vi "metronome.vi"(8 "error in (no error)":errorcluster, 11 "Refnum in":T1) -> (0 "error out":errorcluster)   [LabVIEW 2014]
uses:
  Controls/FPGA Reference.ctl
  Controls/Application Data.vi
  <vilib>/Utility/error.llb/Error Cluster From Error Code.vi
  <vilib>/rvi/errors/niLvFpgaAdjustHostInterfaceError.vi
  <vilib>/rvi/interface/nirviReadWriteControl/nirviReadWriteControl.xnode
  <vilib>/rvi/interface/Simulation/niFpgaSimulationCallBeginRW.vi
  NiFpgaLv.dll
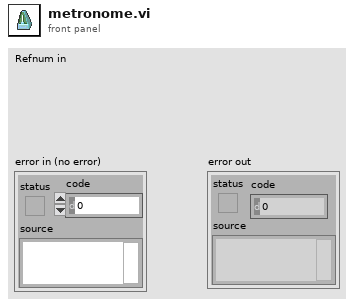
[diagram p1: front panel]
types:
  T1 = typedef "FPGA Reference.ctl" = refnum<k20>
  T2 = cluster{"LED 0":bool, "LED 1":bool, "LED 2":bool, "LED 3":bool}
  T3 = typedef "playback state.ctl" = enum16{"Load File", "Save File", "Play", "Record", "Stop", "Rewind"}
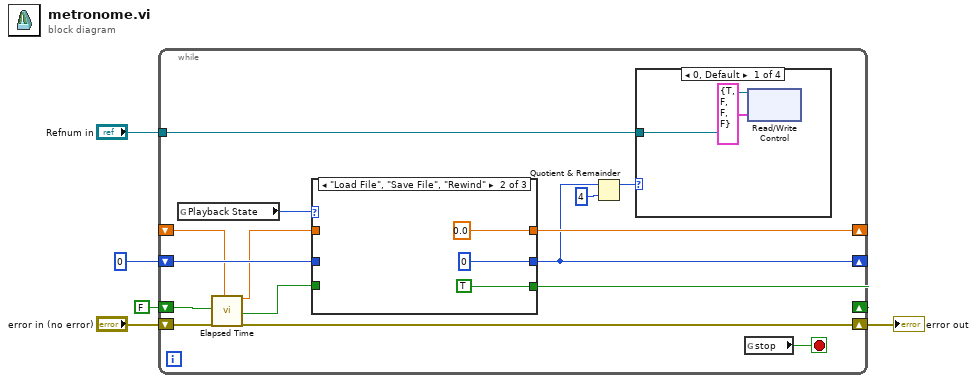
[diagram p0: block diagram]
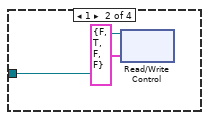
[diagram p2: hidden frame]
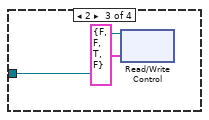
[diagram p3: hidden frame]
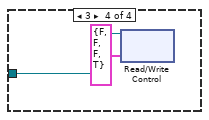
[diagram p4: hidden frame]
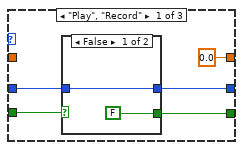
[diagram p5: hidden frame]
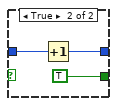
[diagram p6: hidden frame]
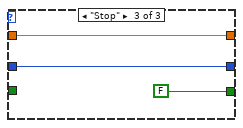
[diagram p7: hidden frame]
diagram:
  n1 = while {
    shift-right: [w11] -> _
    shift-left: 0 -> [w17]
    shift-right: [w16] -> _
    shift-left: FALSE -> [w15]
    shift-right: [w13] -> _
    shift-left: _ -> [w12]
    tunnel: "Refnum in" -> [w8]
    shift-right: [w6] -> w2
    shift-left: "error in (no error)" -> [w7]
    stop <- w20 stop-if-true
    n2 = global read "Application Data.vi" "Playback State"() -> (w19:T3)
    n3 = call "Elapsed Time"("Reset"=w15, "error in (no error)"=w7, "Set Start Time (s)"=w12) -> ("Present (s)"=w14:dbl, "Time has Elapsed"=w18:bool, "error out"=w6:errorcluster)  [unwired: 9 in, 5 out]
    n4 = case shown="\"Load File\", \"Save File\", \"Rewind\"" w19 {
      tunnel: w18 -> [w31 _ _]
      tunnel: w17 -> [w33 _ w42]
      tunnel: [w32 0 w42] -> w11
      tunnel: [w30 TRUE FALSE] -> w16
      tunnel: w14 -> [_ _ w44]
      tunnel: [0.0 ("Present (s)") 0.0 ("Present (s)") w44] -> w13
      frame "Play", "Record" {
        n5 = case shown="False" w31 {
          tunnel: w33 -> [w35 w38]
          tunnel: [w35 w37] -> w32
          tunnel: [FALSE TRUE] -> w30
          frame False {
          }
          frame True {
            n6 = Increment(x=w38) -> (x+1=w37:i32)
          }
        }
      }
      frame "Load File", "Save File", "Rewind" {
      }
      frame "Stop" {
      }
    }
    n7 = Quotient & Remainder(x=w11, y=4) -> (x-y*floor(x/y)=w9:i32)  [unwired: 1 out]
    n8 = case shown="0, Default" w9 {
      tunnel: w8 -> [w22 w24 w26 w28]
      frame 0, Default {
        n9 = xnode "Read/Write Control"("FPGA VI Reference In"=w22, "LEDs"=T2 {"LED 0"=TRUE, "LED 1"=FALSE, "LED 2"=FALSE, "LED 3"=FALSE}) -> ()  [unwired: 1 in, 2 out]
      }
      frame 1 {
        n10 = xnode "Read/Write Control"("FPGA VI Reference In"=w24, "LEDs"=T2 {"LED 0"=FALSE, "LED 1"=TRUE, "LED 2"=FALSE, "LED 3"=FALSE}) -> ()  [unwired: 1 in, 2 out]
      }
      frame 2 {
        n11 = xnode "Read/Write Control"("FPGA VI Reference In"=w26, "LEDs"=T2 {"LED 0"=FALSE, "LED 1"=FALSE, "LED 2"=TRUE, "LED 3"=FALSE}) -> ()  [unwired: 1 in, 2 out]
      }
      frame 3 {
        n12 = xnode "Read/Write Control"("FPGA VI Reference In"=w28, "LEDs"=T2 {"LED 0"=FALSE, "LED 1"=FALSE, "LED 2"=FALSE, "LED 3"=TRUE}) -> ()  [unwired: 1 in, 2 out]
      }
    }
    n13 = global read "Application Data.vi" "stop"() -> (w20:bool)
  }
  "error out" <- w2
